vi "Control Paths.vi"(11 "VolatusControlsList in":refnum<class "VolatusControlsList.lvclass">) -> (2 "Control Paths":path[](array[path]))   [LabVIEW 2020, in "VolatusGUIControls.lvlib" / "VolatusControlsList.lvclass"]
uses:
  VolatusControlsList.lvclass
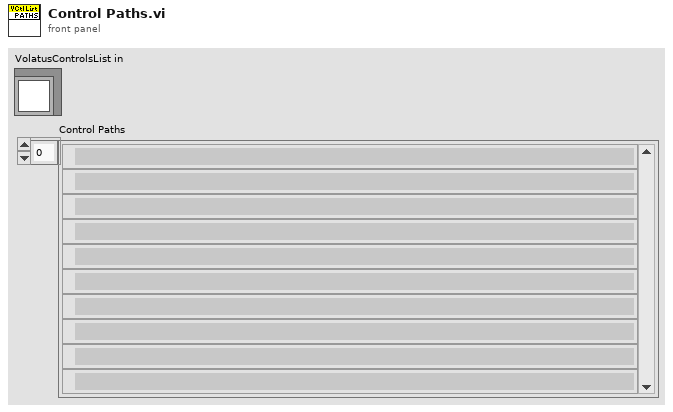
[diagram p1: front panel]
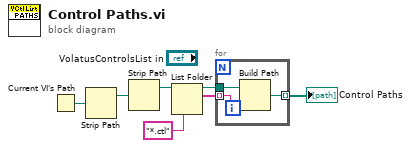
[diagram p0: block diagram]
diagram:
  n1 = Current VI's Path() -> (path=w7:path)
  n2 = Strip Path(path=w7) -> (stripped path=w6:path)  [unwired: 1 out]
  n3 = Strip Path(path=w6) -> (stripped path=w1:path)  [unwired: 1 out]
  n4 = List Folder(path=w1, pattern="*.ctl") -> (path out=w4:path, filenames=w3:string[])  [unwired: 2 in, 2 out]
  n5 = for {
    tunnel: w4 -> [w10]
    tunnel: w3 -> [w9] mode=indexing
    tunnel: [w8] -> w2 mode=indexing
    n6 = Build Path(base path=w10, name or relative path=w9) -> (appended path=w8:path)
  }
  "Control Paths" <- w2
